vi "face-recognition.vi"() -> ()   [LabVIEW 2016]
uses:
  <vilib>/userdefined/High Color/IMAQdx.ctl
  <vilib>/vision/driver/NI_Vision_Acquisition_Software.lvlib
  <vilib>/vision/NI_Vision_Development_Module.lvlib
panel:
  in  "Settings 3":T1={"Algorithm"=2, "Number of Matches Requested"=1, "Minimum Match Score"=800.0, "SubPixel Accuracy"=TRUE, "Rotation Angle Ranges"=[], "Show Search Area"=FALSE, "Show Result"=TRUE} {"Rotation Angle Ranges"."End" format="%.1f"; "Rotation Angle Ranges"."Start" format="%.1f"; "Minimum Match Score" min=0 max=1000 format="%.2f"; "Number of Matches Requested" min=1; "Algorithm" items=["All", "Low Discrepancy Sampling", "Grayscale Value Pyramid", "Gradients Pyramid"]}
  out "Eyes":T2(plugin-control)
  in  "?":u16(ring) items=["Face", "Nose", "Eyes"]
  in  "Settings 2":T1={"Algorithm"=2, "Number of Matches Requested"=1, "Minimum Match Score"=800.0, "SubPixel Accuracy"=TRUE, "Rotation Angle Ranges"=[], "Show Search Area"=FALSE, "Show Result"=TRUE} {"Rotation Angle Ranges"."End" format="%.1f"; "Rotation Angle Ranges"."Start" format="%.1f"; "Minimum Match Score" min=0 max=1000 format="%.2f"; "Number of Matches Requested" min=1; "Algorithm" items=["All", "Low Discrepancy Sampling", "Grayscale Value Pyramid", "Gradients Pyramid"]}
  out "Nose":T2(plugin-control)
  in  "Settings":T1={"Algorithm"=2, "Number of Matches Requested"=1, "Minimum Match Score"=800.0, "SubPixel Accuracy"=TRUE, "Rotation Angle Ranges"=[], "Show Search Area"=FALSE, "Show Result"=TRUE} {"Rotation Angle Ranges"."End" format="%.1f"; "Rotation Angle Ranges"."Start" format="%.1f"; "Minimum Match Score" min=0 max=1000 format="%.2f"; "Number of Matches Requested" min=1; "Algorithm" items=["All", "Low Discrepancy Sampling", "Grayscale Value Pyramid", "Gradients Pyramid"]}
  in  "Search":bool
  in  "?":bool
  out "Face":T2(plugin-control)
  out "Image":T2(plugin-control)
  in  "Session In":T3
  # "Description:\n\nThis program uses pattern recognition to identify the face, nose, and eyes of the user.\n\nInstructions:\n\n1. Run the program.\n\n2. Select your camera in the Session In menu.\n\n3. Select the facial feature you want to identify using the menu ring.\n\n4. Draw a box around the feature in the Image display.\n\n5. Repeat steps 3-4 for the remaining two features.\n\n6. Press the Search button.\n\n7. View the pattern recognition results in the Image display.\n\n8. Press the STOP button to terminate the program."
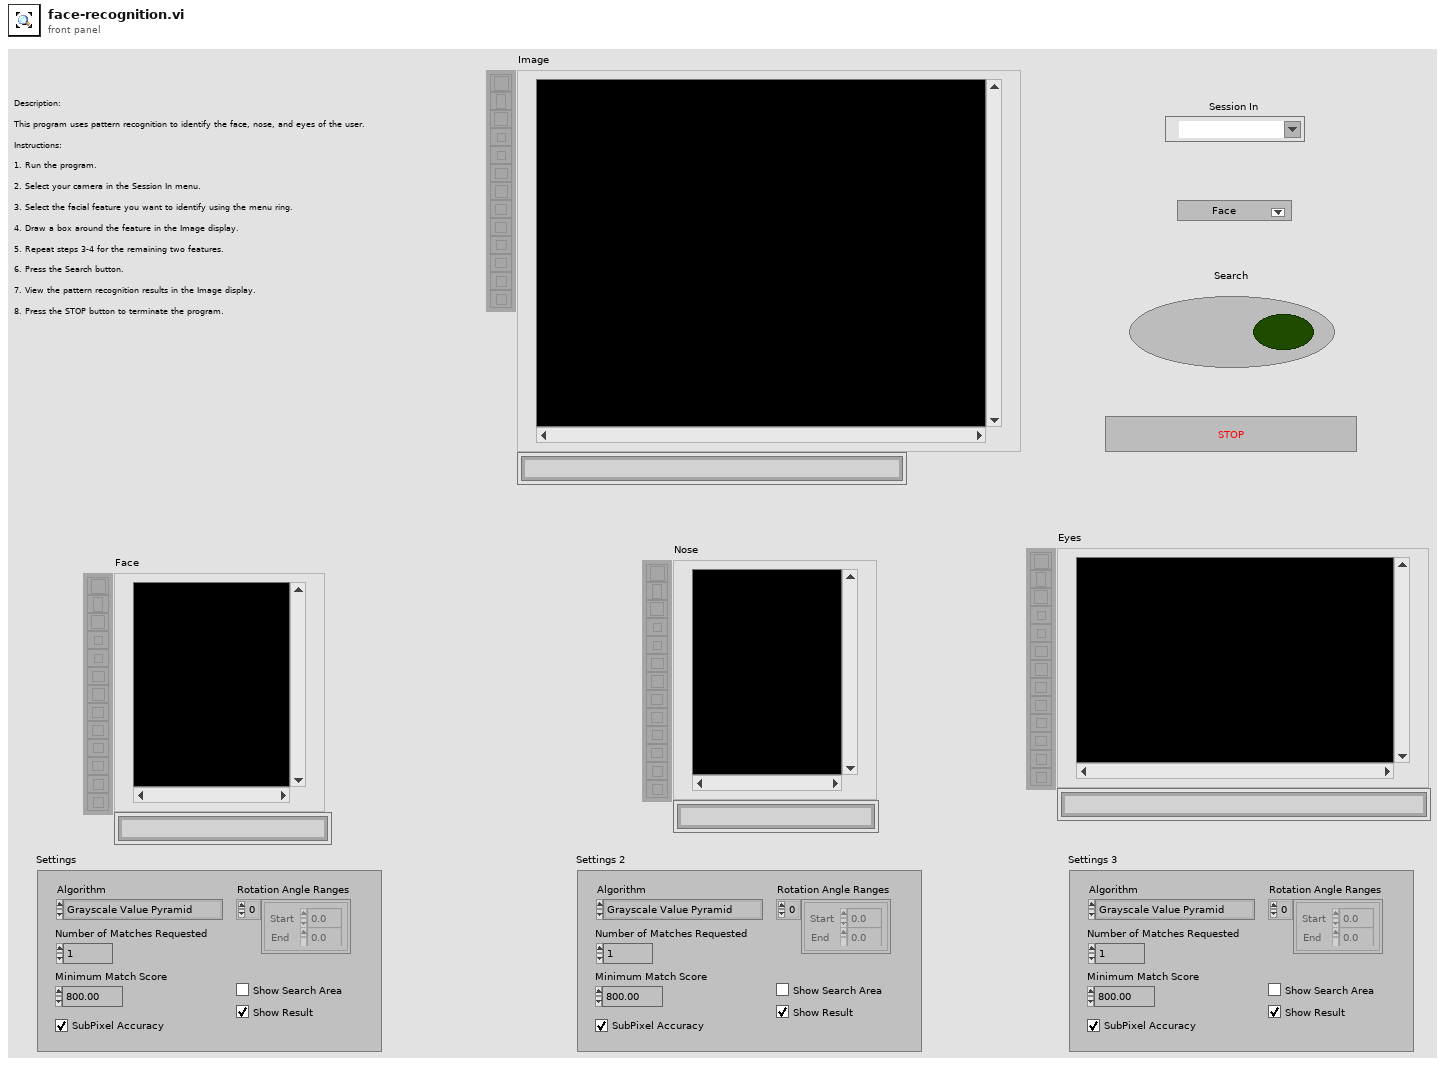
[diagram p1: front panel]
types:
  T1 = cluster{"Algorithm":i32, "Number of Matches Requested":i32, "Minimum Match Score":sgl, "SubPixel Accuracy":bool, "Rotation Angle Ranges":cluster{"Start":sgl, "End":sgl}[], "Show Search Area":bool, "Show Result":bool}
  T2 = typedef "IMAQ Image.ctl" = refnum<image>
  T3 = typedef "IMAQdx.ctl" = refnum<k21>
  T4 = typedef "Image Type" = u32
  T5 = cluster{"Position":cluster{"x":sgl, "y":sgl}, "Angle":sgl, "Scale":sgl, "Score":sgl, "Bounding Box":cluster{"x":sgl, "y":sgl}[]}[]
  T6 = cluster{"Matches (pixel)[0]":cluster{"Position":cluster{"x":sgl, "y":sgl}, "Angle":sgl, "Scale":sgl, "Score":sgl, "Bounding Box":cluster{"x":sgl, "y":sgl}[]}, "Matches (pixel)[1]":cluster{"Position":cluster{"x":sgl, "y":sgl}, "Angle":sgl, "Scale":sgl, "Score":sgl, "Bounding Box":cluster{"x":sgl, "y":sgl}[]}, "Matches (pixel)[2]":cluster{"Position":cluster{"x":sgl, "y":sgl}, "Angle":sgl, "Scale":sgl, "Score":sgl, "Bounding Box":cluster{"x":sgl, "y":sgl}[]}, "Matches (pixel)[3]":cluster{"Position":cluster{"x":sgl, "y":sgl}, "Angle":sgl, "Scale":sgl, "Score":sgl, "Bounding Box":cluster{"x":sgl, "y":sgl}[]}, "Matches (pixel)[4]":cluster{"Position":cluster{"x":sgl, "y":sgl}, "Angle":sgl, "Scale":sgl, "Score":sgl, "Bounding Box":cluster{"x":sgl, "y":sgl}[]}, "Matches (pixel)[5]":cluster{"Position":cluster{"x":sgl, "y":sgl}, "Angle":sgl, "Scale":sgl, "Score":sgl, "Bounding Box":cluster{"x":sgl, "y":sgl}[]}, "Matches (pixel)[6]":cluster{"Position":cluster{"x":sgl, "y":sgl}, "Angle":sgl, "Scale":sgl, "Score":sgl, "Bounding Box":cluster{"x":sgl, "y":sgl}[]}, "Matches (pixel)[7]":cluster{"Position":cluster{"x":sgl, "y":sgl}, "Angle":sgl, "Scale":sgl, "Score":sgl, "Bounding Box":cluster{"x":sgl, "y":sgl}[]}, "Matches (pixel)[8]":cluster{"Position":cluster{"x":sgl, "y":sgl}, "Angle":sgl, "Scale":sgl, "Score":sgl, "Bounding Box":cluster{"x":sgl, "y":sgl}[]}}
  T7 = cluster{"Position":cluster{"x":sgl, "y":sgl}, "Angle":sgl, "Scale":sgl, "Score":sgl, "Bounding Box":cluster{"x":sgl, "y":sgl}[]}
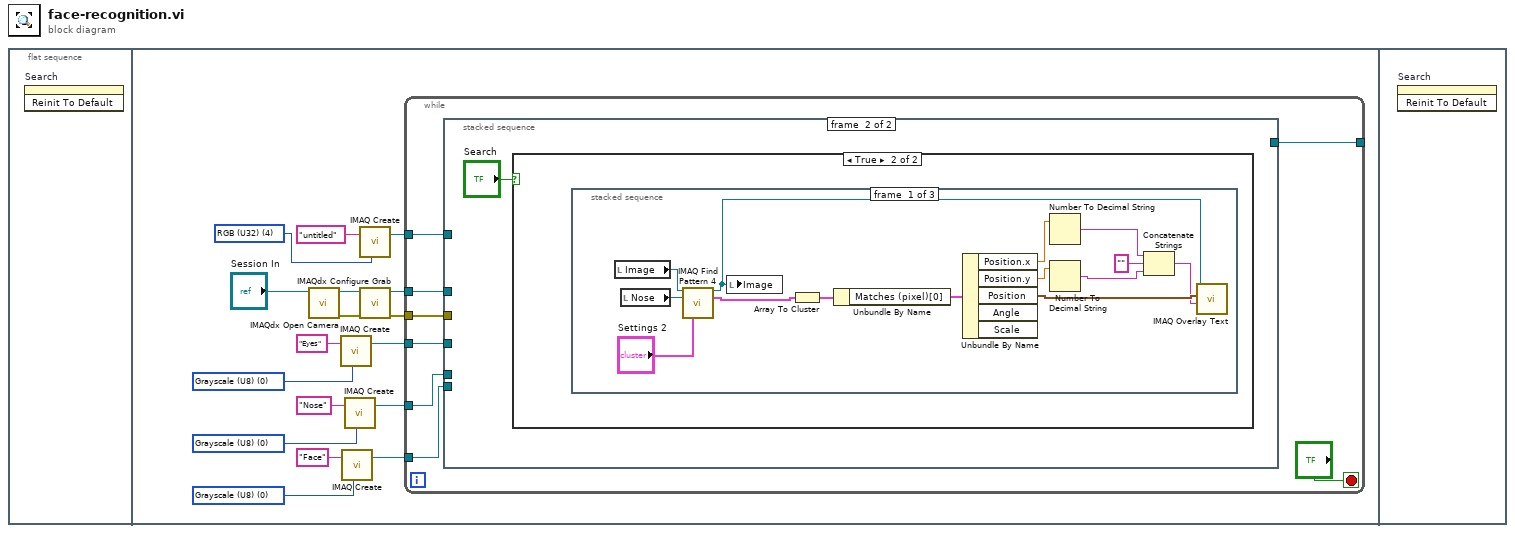
[diagram p0: block diagram]
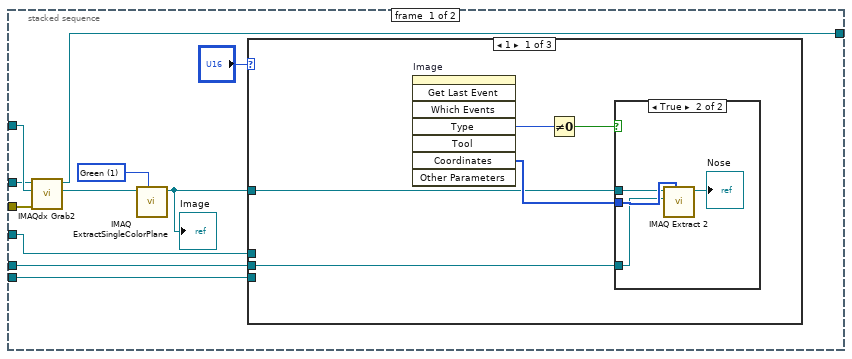
[diagram p2: hidden frame]
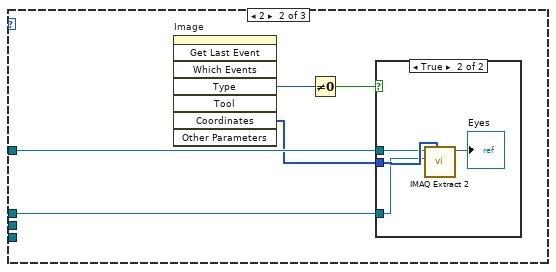
[diagram p4: hidden frame]
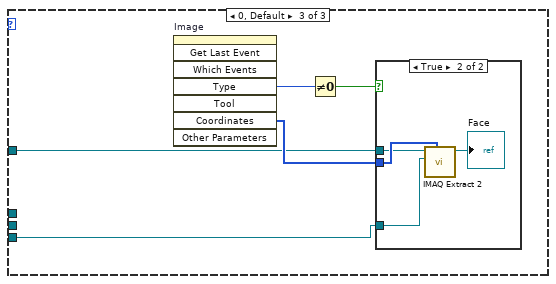
[diagram p6: hidden frame]
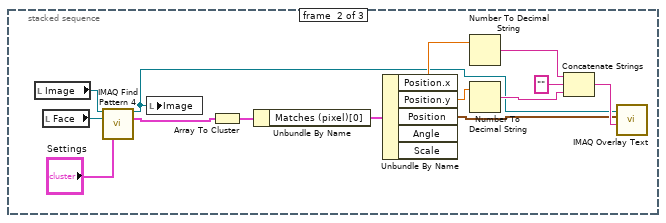
[diagram p9: hidden frame]
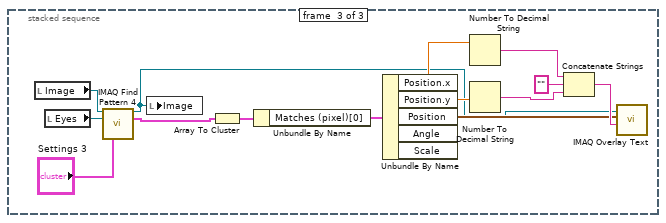
[diagram p10: hidden frame]
diagram:
  n1 = flat-sequence {
    frame #0 {
      n2 = invoke on="Search" class="Bool (strict)" method="Reinit To Default"() -> ()  [unwired: 3 in, 3 out]
    }
    frame #1 {
      w2 = T4 0 items=["Grayscale (U8)", "Grayscale (I16)", "Grayscale (SGL)", "Complex (CSG)", "RGB (U32)", "HSL (U32)", "RGB (U64)", "Grayscale (U16)"] ("Image Type")
      w6 = T4 0 items=["Grayscale (U8)", "Grayscale (I16)", "Grayscale (SGL)", "Complex (CSG)", "RGB (U32)", "HSL (U32)", "RGB (U64)", "Grayscale (U16)"] ("Image Type")
      w8 = T4 0 items=["Grayscale (U8)", "Grayscale (I16)", "Grayscale (SGL)", "Complex (CSG)", "RGB (U32)", "HSL (U32)", "RGB (U64)", "Grayscale (U16)"] ("Image Type")
      w13 = T4 4 items=["Grayscale (U8)", "Grayscale (I16)", "Grayscale (SGL)", "Complex (CSG)", "RGB (U32)", "HSL (U32)", "RGB (U64)", "Grayscale (U16)"] ("Image Type")
      n3 = call <vilib>:"IMAQdx Open Camera.vi"("Session In"="Session In") -> ("error out"=w16:errorcluster, "Session Out"=w17:T3)  [unwired: 9 in]
      n4 = call "IMAQ Create"("Image Name"="Eyes", "Image Type"=w2) -> ("New Image"=w1:T2)  [unwired: 3 in, 1 out]
      n5 = call "IMAQ Create"("Image Name"="Face", "Image Type"=w8) -> ("New Image"=w7:T2)  [unwired: 3 in, 1 out]
      n6 = call "IMAQ Create"("Image Name"="Nose", "Image Type"=w6) -> ("New Image"=w4:T2)  [unwired: 3 in, 1 out]
      n7 = call "IMAQ Create"("Image Name"="untitled", "Image Type"=w13) -> ("New Image"=w10:T2)  [unwired: 3 in, 1 out]
      n8 = call <vilib>:"IMAQdx Configure Grab.vi"("error in"=w16, "Session In"=w17) -> ("error out"=w11:errorcluster, "Session Out"=w12:T3)  [unwired: 8 in]
      n9 = while {
        tunnel: w12 -> [w25]
        tunnel: w11 -> [w24]
        tunnel: w10 -> [w23]
        tunnel: w7 -> [w22]
        tunnel: [w20] -> _
        tunnel: w4 -> [w19]
        tunnel: w1 -> [w18]
        stop <- "?" stop-if-true
        n10 = stacked-sequence {
          tunnel: w25 -> [w33 _]
          tunnel: w24 -> [w32 _]
          tunnel: w23 -> [w34 _]
          tunnel: w22 -> [w29 _]
          tunnel: [w31 _] -> w20
          tunnel: w19 -> [w27 _]
          tunnel: w18 -> [w26 _]
          frame #0 {
            w36 = 1 items=["Red", "Green", "Blue", "Hue", "Saturation", "Luminance", "Value", "Intensity"] ("Color Plane")
            n11 = call <vilib>:"IMAQdx Grab2.vi"("error in"=w32, "Image In"=w34, "Session In"=w33) -> ("Image Out"=w35:T2, "Session Out"=w31:T3)  [unwired: 5 in, 2 out]
            n12 = call "IMAQ ExtractSingleColorPlane"("Color Plane"=w36, "Image Src"=w35) -> ("Image Dst Out"=w30:T2)  [unwired: 8 in, 1 out]
            "Image" <- w30
            n13 = case shown="1" "?" {
              tunnel: w30 -> [w38 w48 w56]
              tunnel: w29 -> [_ _ w55]
              tunnel: w27 -> [w37 _ _]
              tunnel: w26 -> [_ w49 _]
              frame 1 {
                n14 = invoke on="Image" class="ImageControl" method="Get Last Event"() -> ("Type"=w40:i32, "Coordinates"=w39:i32[])  [unwired: 8 in, 6 out]
                n15 = Not Equal To 0?(x=w40) -> (x != 0?=w41:bool)
                n16 = case shown="True" w41 {
                  tunnel: w39 -> [_ w44]
                  tunnel: w38 -> [_ w43]
                  tunnel: w37 -> [_ w42]
                  frame False {
                  }
                  frame True {
                    n17 = call "IMAQ Extract 2"("Optional Rectangle"=w44, "Image Dst"=w42, "Image Src"=w43) -> ("Image Dst Out"=→"Nose":T2)  [unwired: 7 in, 1 out]
                  }
                }
              }
              frame 2 {
                n18 = invoke on="Image" class="ImageControl" method="Get Last Event"() -> ("Type"=w47:i32, "Coordinates"=w46:i32[])  [unwired: 8 in, 6 out]
                n19 = Not Equal To 0?(x=w47) -> (x != 0?=w50:bool)
                n20 = case shown="True" w50 {
                  tunnel: w46 -> [_ w53]
                  tunnel: w49 -> [_ w52]
                  tunnel: w48 -> [_ w51]
                  frame False {
                  }
                  frame True {
                    n21 = call "IMAQ Extract 2"("Optional Rectangle"=w53, "Image Dst"=w52, "Image Src"=w51) -> ("Image Dst Out"=→"Eyes":T2)  [unwired: 7 in, 1 out]
                  }
                }
              }
              frame 0, Default {
                n22 = invoke on="Image" class="ImageControl" method="Get Last Event"() -> ("Type"=w57:i32, "Coordinates"=w59:i32[])  [unwired: 8 in, 6 out]
                n23 = Not Equal To 0?(x=w57) -> (x != 0?=w58:bool)
                n24 = case shown="True" w58 {
                  tunnel: w59 -> [_ w63]
                  tunnel: w56 -> [_ w61]
                  tunnel: w55 -> [_ w60]
                  frame False {
                  }
                  frame True {
                    n25 = call "IMAQ Extract 2"("Optional Rectangle"=w63, "Image Dst"=w60, "Image Src"=w61) -> ("Image Dst Out"=→"Face":T2)  [unwired: 7 in, 1 out]
                  }
                }
              }
            }
          }
          frame #1 {
            n26 = case shown="True" "Search" {
              frame False {
              }
              frame True {
                n27 = stacked-sequence {
                  frame #0 {
                    n28 = local read "Image"() -> (w78:T2)
                    n29 = local read "Nose"() -> (w77:T2)
                    n30 = call "IMAQ Find Pattern 4"("Image"=w78, "Template"=w77, "Settings"="Settings 2") -> ("Image Out"=w76:T2, "Matches (pixel)"=w67:T5)  [unwired: 6 in, 5 out]
                    n31 = local write "Image"(w76) -> ()
                    n32 = Array To Cluster(array=w67) -> (cluster=w68:T6)
                    n33 = Unbundle By Name(w68) -> ("Matches (pixel)[0]"=w69:T7)
                    n34 = Unbundle By Name(w69) -> ("Position.x"=w71:sgl, "Position.y"=w72:sgl, "Position"=w70:cluster{"x":sgl, "y":sgl})  [unwired: 2 out]
                    n35 = Number To Decimal String(number=w71) -> (decimal integer string=w73:string)  [unwired: 1 in]
                    n36 = Number To Decimal String(number=w72) -> (decimal integer string=w74:string)  [unwired: 1 in]
                    n37 = Concatenate Strings(w73, "" ("string"), w74) -> (w66:string)
                    n38 = call "IMAQ Overlay Text"("String"=w66, "Origin"=w70, "Image"=w76) -> ()  [unwired: 7 in, 2 out]
                  }
                  frame #1 {
                    n39 = local read "Image"() -> (w79:T2)
                    n40 = local read "Face"() -> (w80:T2)
                    n41 = call "IMAQ Find Pattern 4"("Image"=w79, "Template"=w80, "Settings"="Settings") -> ("Image Out"=w81:T2, "Matches (pixel)"=w90:T5)  [unwired: 6 in, 5 out]
                    n42 = local write "Image"(w81) -> ()
                    n43 = Array To Cluster(array=w90) -> (cluster=w89:T6)
                    n44 = Unbundle By Name(w89) -> ("Matches (pixel)[0]"=w88:T7)
                    n45 = Unbundle By Name(w88) -> ("Position.x"=w86:sgl, "Position.y"=w85:sgl, "Position"=w87:cluster{"x":sgl, "y":sgl})  [unwired: 2 out]
                    n46 = Number To Decimal String(number=w86) -> (decimal integer string=w84:string)  [unwired: 1 in]
                    n47 = Number To Decimal String(number=w85) -> (decimal integer string=w83:string)  [unwired: 1 in]
                    n48 = Concatenate Strings(w84, "" ("string"), w83) -> (w91:string)
                    n49 = call "IMAQ Overlay Text"("String"=w91, "Origin"=w87, "Image"=w81) -> ()  [unwired: 7 in, 2 out]
                  }
                  frame #2 {
                    n50 = local read "Image"() -> (w94:T2)
                    n51 = local read "Eyes"() -> (w95:T2)
                    n52 = call "IMAQ Find Pattern 4"("Image"=w94, "Template"=w95, "Settings"="Settings 3") -> ("Image Out"=w96:T2, "Matches (pixel)"=w104:T5)  [unwired: 6 in, 5 out]
                    n53 = local write "Image"(w96) -> ()
                    n54 = Array To Cluster(array=w104) -> (cluster=w103:T6)
                    n55 = Unbundle By Name(w103) -> ("Matches (pixel)[0]"=w102:T7)
                    n56 = Unbundle By Name(w102) -> ("Position.x"=w100:sgl, "Position.y"=w99:sgl, "Position"=w101:cluster{"x":sgl, "y":sgl})  [unwired: 2 out]
                    n57 = Number To Decimal String(number=w100) -> (decimal integer string=w98:string)  [unwired: 1 in]
                    n58 = Number To Decimal String(number=w99) -> (decimal integer string=w93:string)  [unwired: 1 in]
                    n59 = Concatenate Strings(w98, "" ("string"), w93) -> (w105:string)
                    n60 = call "IMAQ Overlay Text"("String"=w105, "Origin"=w101, "Image"=w96) -> ()  [unwired: 7 in, 2 out]
                  }
                }
              }
            }
          }
        }
      }
    }
    frame #2 {
      n61 = invoke on="Search" class="Bool (strict)" method="Reinit To Default"() -> ()  [unwired: 3 in, 3 out]
    }
  }
